vi "Auton Builder.vi"() -> ()   [LabVIEW 2017]
uses:
  Typedef/Field Settings.ctl
  Typedef/Robot Settings.ctl
  Typedef/Single Sequence.ctl
  Typedef/Sequence Command.ctl
  Typedef/Plate Arrangement.ctl
  Typedef/String Commands.ctl
  <vilib>/Utility/miscctls.llb/LVRowAndColumnTypeDef.ctl
  <vilib>/Analysis/coordinate.llb/2D Cartesian Coordinate Rotation (Array).vi
  <vilib>/Analysis/coordinate.llb/2D Cartesian Coordinate Shift (Array).vi
  <vilib>/Rock Robotics/Network Tables/NT Write Variant.vi
  <vilib>/Analysis/NI_AALPro.lvlib
panel:
  in  "Stop?":bool
  in  "Tab Control":enum32{"Builder", "Raw Sequence", "Settings"}(tab)
  in  "Index?":i32
  out "Issue:":string
  in  "Drive Time":bool
  in  "Other Commands":T1
  out "Current Command":string
  in  "Open":bool
  in  "Save":bool
  in  "Reset":bool
  out "Sequence Ok?":bool
  in  "Send to Robot":bool
  in  "Simulate":bool
  in  "Drive Path":bool
  in  "Turn Degrees":bool
  in  "Sequence Number":u32
  in  "Name":string
  in  "Plate Arrangement":T2={"LR*"=TRUE, "LL*"=TRUE, "RL*"=TRUE, "RR*"=TRUE}
  in  "Add":bool
  in  "Sequence":i32(listbox)
  in  "Right":bool
  in  "Mid":bool
  in  "Left":bool
  out "Field Half":cluster{dbl[], dbl[]}[](graph)
  in  "Cancel":bool
  in  "Auton Sequence":T3[](array[typedef])
  in  "Path Folder":path
  in  "Robot IP":string="roboRIO-3005-FRC.local"
  out "Connected?":bool
  in  "Field Settings":T5={"Exchange Left"=102.0, "Exchange Right"=150.0, "Power Cube Zone Left"=139.5, "Power Cube Zone Right"=139.5, "Switch Left"=85.25, "Switch Right"=85.25, "Switch Front"=140.0, "Switch Back"=196.0, "Platform Left"=95.25, "Platform Right"=95.25, "Platform Front"=261.47, "Slalom Depth"=235.235}
  in  "Robot Settings":T6={"Width"=34.0, "Length"=39.0} caption="Robot Settings w/ Bumpers"
  # "LEFT"
  # "FAR"
  # "NEAR"
  # "RIGHT"
  # "Commands"
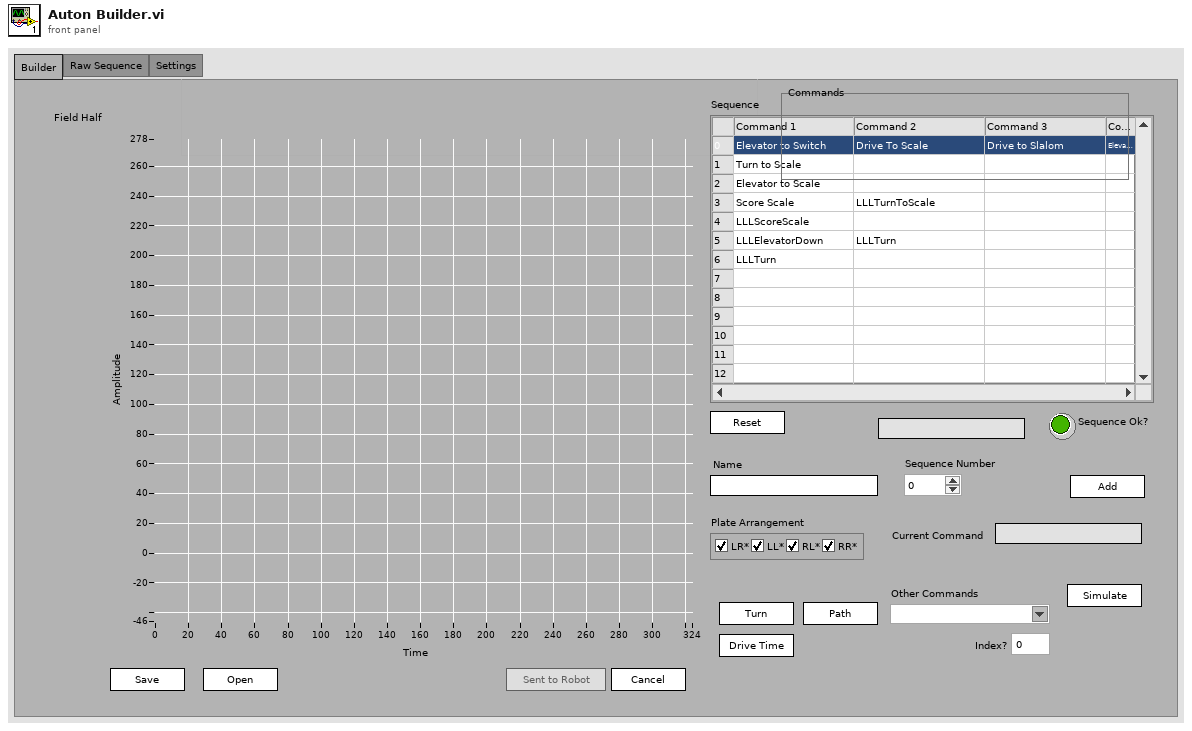
[diagram p1: front panel]
types:
  T1 = typedef "String Commands.ctl" = string
  T2 = typedef "Plate Arrangement.ctl" = cluster{"LR*":bool, "LL*":bool, "RL*":bool, "RR*":bool}
  T3 = typedef "Single Sequence.ctl" = cluster{"Sequence Array":T4[]}
  T4 = typedef "Sequence Command.ctl" = cluster{"Sequence Name":string, "Plate Arrangement":T2, "Command Name":string, "Data":variant, "Sequence Number":u32}
  T5 = typedef "Field Settings.ctl" = cluster{"Exchange Left":dbl, "Exchange Right":dbl, "Power Cube Zone Left":dbl, "Power Cube Zone Right":dbl, "Switch Left":dbl, "Switch Right":dbl, "Switch Front":dbl, "Switch Back":dbl, "Platform Left":dbl, "Platform Right":dbl, "Platform Front":dbl, "Slalom Depth":dbl}
  T6 = typedef "Robot Settings.ctl" = cluster{"Width":dbl, "Length":dbl}
  T7 = typedef "LVRowAndColumnTypeDef.ctl" = cluster{"Row":i32, "Column":i32}
  T8 = cluster{"Auton Sequence":T3[], "Field Half":cluster{dbl[], dbl[]}[], "Current Command":T4, "Robot Position":cluster{"x":dbl, "y":dbl}, "Theta":dbl, "y position":dbl, "Active Cell":T7, "Robot Index":i32, "Sequence OK?":bool, "Start Position":cluster{"x":dbl, "y":dbl}, "Field Selection":string, "Simulation Index":i32, "Sim Robot Index":i32, "Active Path":path, "Load Index":i32, "Graph Index":i32}
  T9 = typedef "LVPoint32TypeDef.ctl" = cluster{"Horizontal":i32, "Vertical":i32}
  T10 = cluster{"Shift":bool, "Ctrl":bool, "Alt":bool, "Cmd":bool, "Opt":bool}
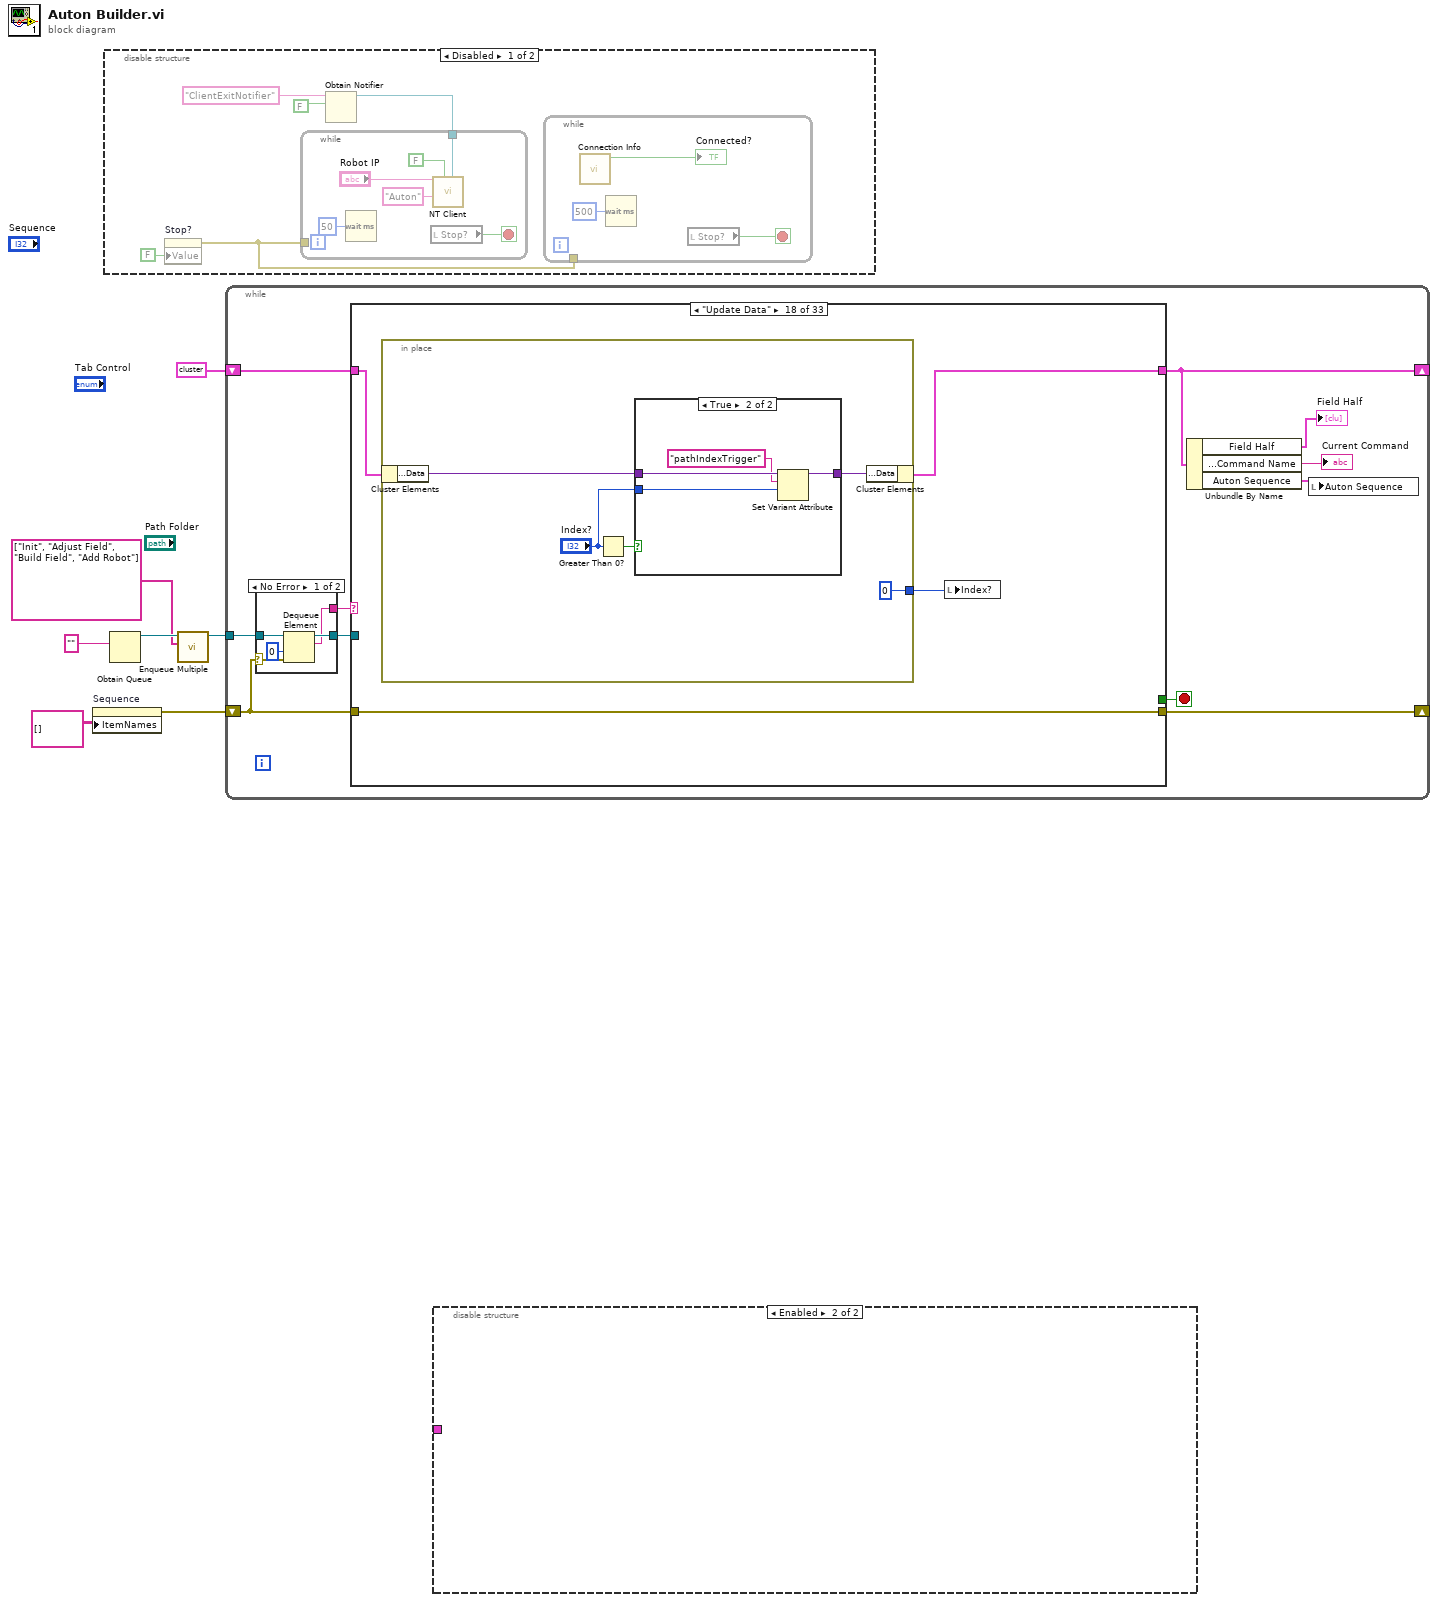
[diagram p0: block diagram]
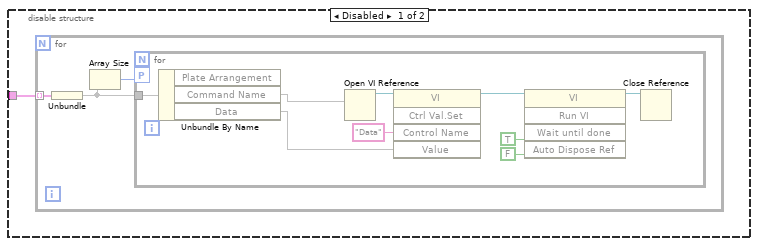
[diagram p3: hidden frame]
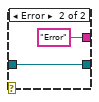
[diagram p4: hidden frame]
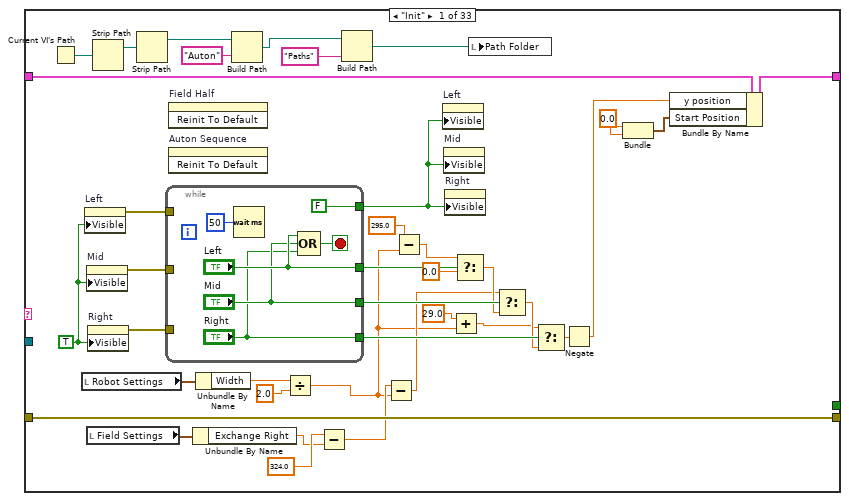
[diagram p5: hidden frame]
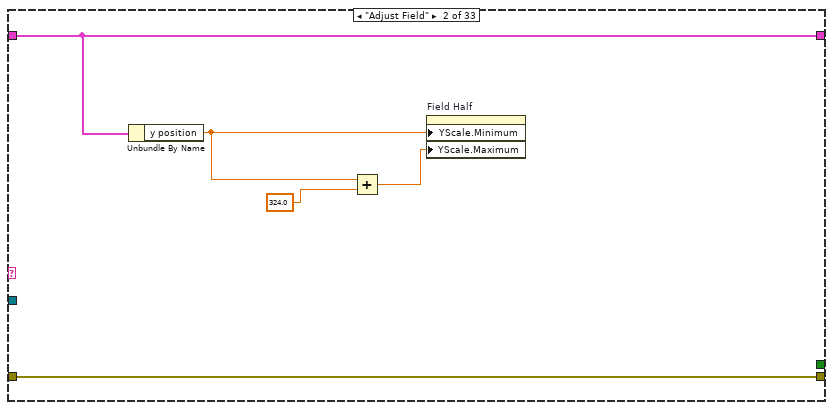
[diagram p6: hidden frame]
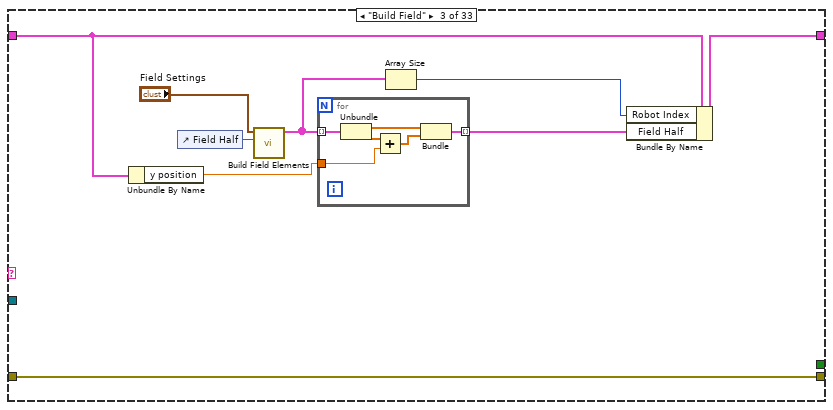
[diagram p7: hidden frame]
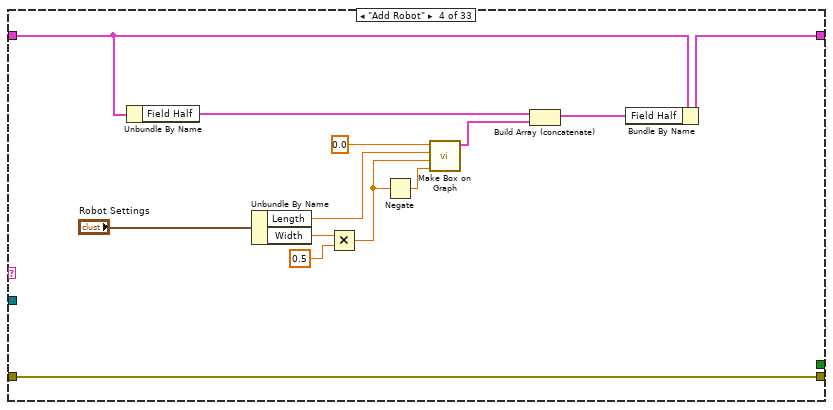
[diagram p8: hidden frame]
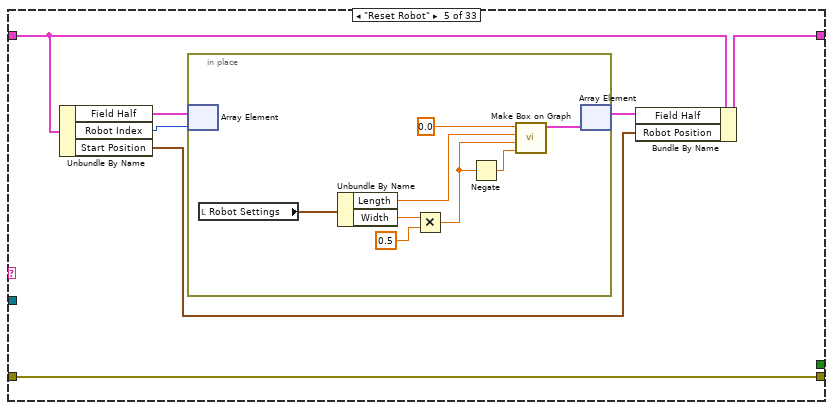
[diagram p9: hidden frame]
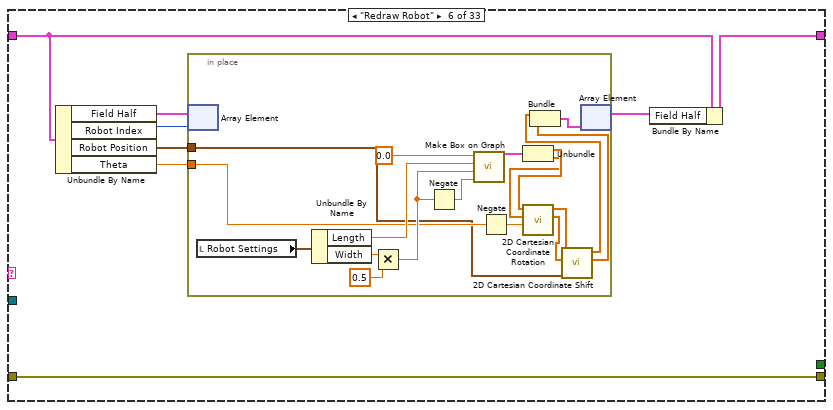
[diagram p10: hidden frame]
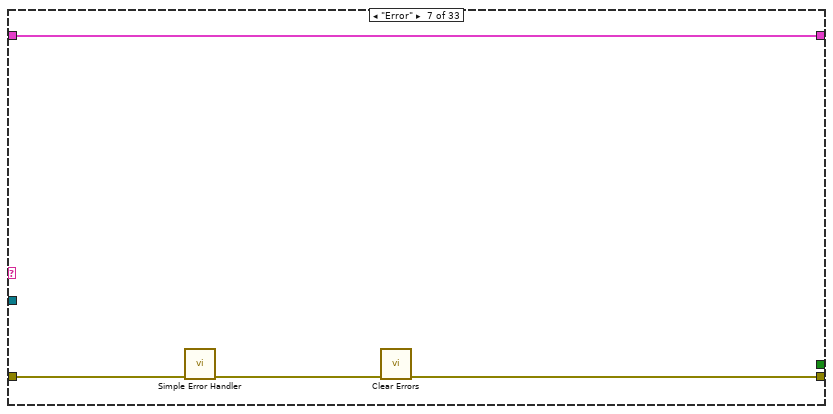
[diagram p11: hidden frame]
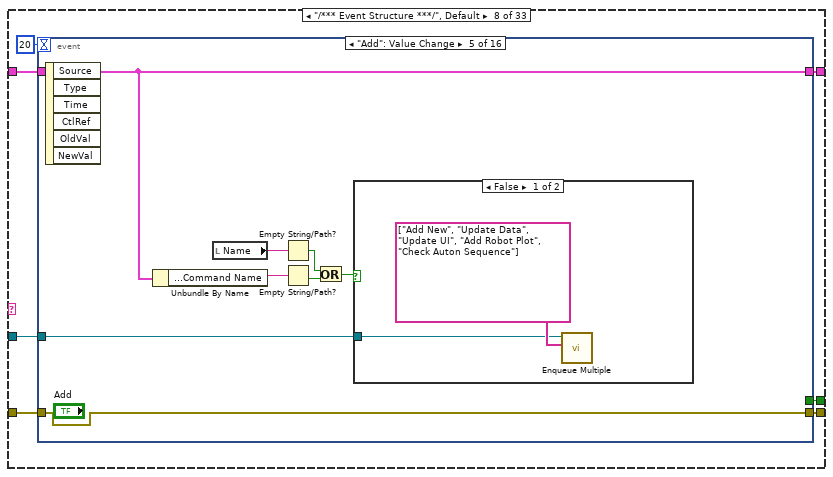
[diagram p12: hidden frame]
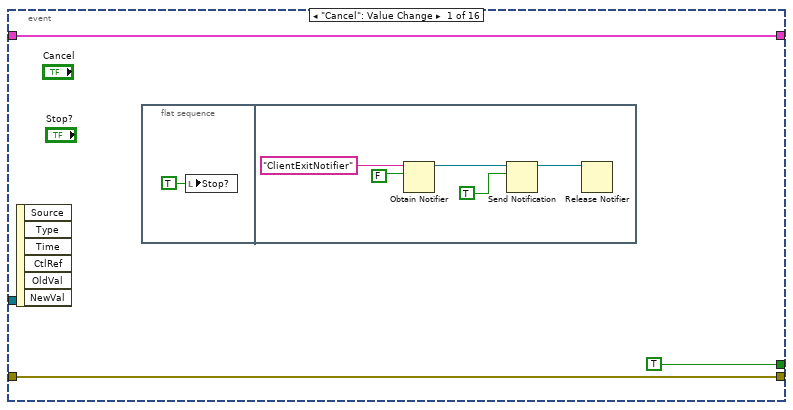
[diagram p13: hidden frame]
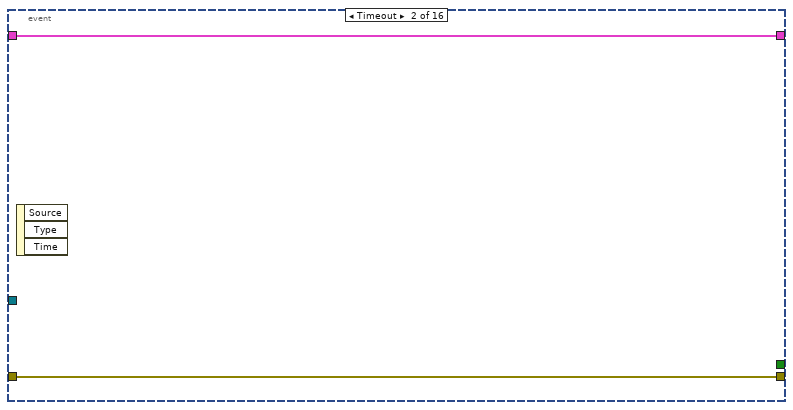
[diagram p14: hidden frame]
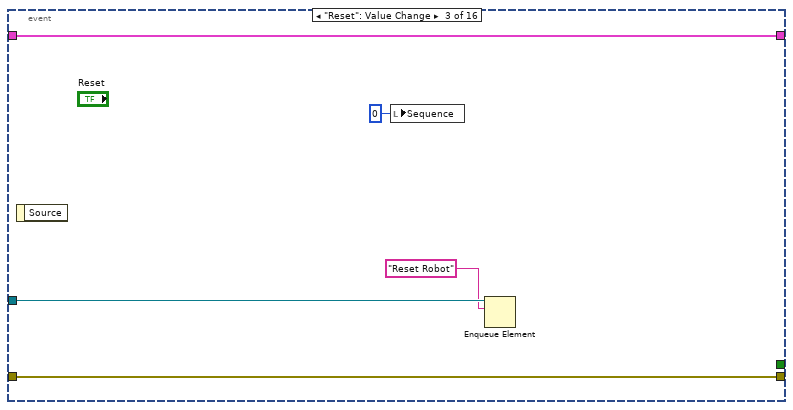
[diagram p15: hidden frame]
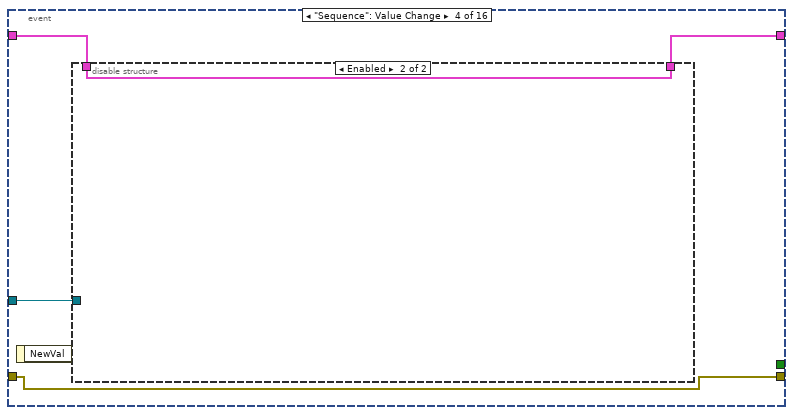
[diagram p16: hidden frame]
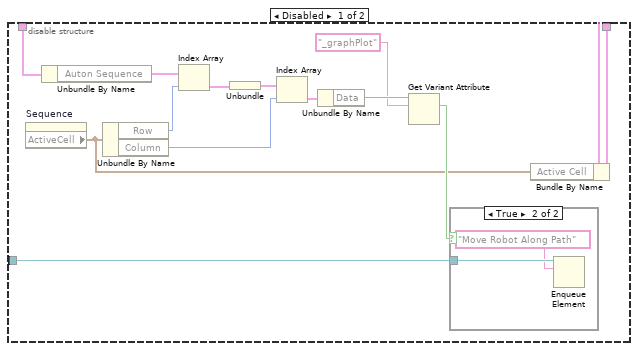
[diagram p17: hidden frame]
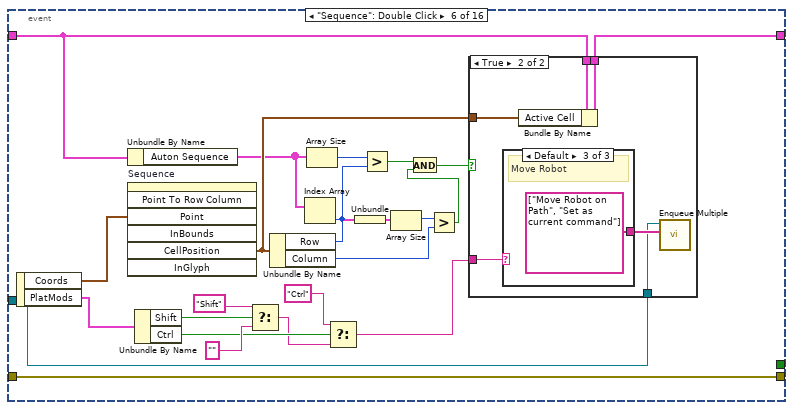
[diagram p20: hidden frame]
diagram:
  n1 = property on="Sequence" class="MCListbox (strict)"("ItemNames"=string[][] [] ("Item Names")) -> (error out=w7:errorcluster)  [unwired: 2 in, 1 out]
  n2 = disable-structure shown="Disabled" {
    frame Disabled {
      n3 = property on="Stop?" class="Bool (strict)"("Value"=FALSE ("Stop?")) -> (error out=w12:errorcluster)  [unwired: 2 in, 1 out]
      n4 = Obtain Notifier(name (unnamed)="ClientExitNotifier", notification data type=FALSE ("Automatic restart")) -> (notifier out=w9:refnum<notifier>)  [unwired: 2 in, 2 out]
      n5 = while {
        tunnel: w9 -> [w20]
        tunnel: w12 -> [_]
        stop <- w17 stop-if-true
        n6 = Wait (ms)(milliseconds to wait=u32 50) -> ()  [unwired: 1 out]
        n7 = local read "Stop?"() -> (w17:bool)
        n8 = call <vilib>:"NT Client.vi"("Cancel Ref"=w20, "Automatic restart"=FALSE, "Client Name"="Auton", "Server IP Address"="Robot IP") -> ()  [unwired: 8 in]
      }
      n9 = while {
        tunnel: w12 -> [_]
        stop <- w13 stop-if-true
        n10 = call <vilib>:"Connection Info.vi"() -> ("Connected"=→"Connected?":bool)  [unwired: 10 in, 1 out]
        n11 = Wait (ms)(milliseconds to wait=u32 500) -> ()  [unwired: 1 out]
        n12 = local read "Stop?"() -> (w13:bool)
      }
    }
    frame Enabled {
    }
  }
  n13 = Obtain Queue(element data type="") -> (queue out=w4:refnum<queue>)  [unwired: 4 in, 2 out]
  n14 = call "Enqueue Multiple.vi"("Array"=string[] ["Init", "Adjust Field", "Build Field", "Add Robot"], "Queue in"=w4) -> ("Queue out"=w3:refnum<queue>)  [unwired: 8 in, 1 out]
  n15 = while {
    shift-right: [w26] -> _
    shift-left: T8 {"Auton Sequence"=[], "Field Half"=[], "Current Command"={"Sequence Name"="", "Plate Arrangement"={"LR*"=FALSE, "LL*"=FALSE, "RL*"=FALSE, "RR*"=FALSE}, "Command Name"="", "Data"=variant, "Sequence Number"=0}, "Robot Position"={"x"=0.0, "y"=0.0}, "Theta"=0.0, "y position"=0.0, "Active Cell"={"Row"=0, "Column"=0}, "Robot Index"=0, "Sequence OK?"=FALSE, "Start Position"={"x"=0.0, "y"=0.0}, "Field Selection"="", "Simulation Index"=0, "Sim Robot Index"=0, "Active Path"=path "", "Load Index"=0, "Graph Index"=0} ("output cluster") -> [w32]
    shift-right: [w28] -> _
    shift-left: w7 -> [w27]
    tunnel: w3 -> [w31]
    stop <- w24 stop-if-true
    n16 = case shown="No Error" w27 {
      selector: w27 -> [w35 _]
      tunnel: w31 -> [w37 w39]
      tunnel: [w36 w39] -> w30
      tunnel: [w34 "Error"] -> w29
      frame No Error {
        n17 = Dequeue Element(queue=w37, timeout in ms (-1)=0, error in (no error)=w35) -> (queue out=w36:refnum<queue>, element=w34:string)  [unwired: 2 out]
      }
      frame Error {
      }
    }
    n18 = case shown="\"Update Data\"" w29 {
      tunnel: [_ _ _ _ _ _ _ w168 _ _ _ _ _ _ _ _ _ _ _ _ _ _ _ _ _ _ _ _ _ _ _ _ _] -> w24
      tunnel: w32 -> [w65 w87 w96 w106 w122 w138 w161 w167 w384 w402 w438 w456 w470 w483 w496 w513 w522 w541 w560 w575 w590 w632 w639 w646 w653 w655 w725 w739 w746 w758 w777 w791 w822]
      tunnel: [w64 w87 w94 w108 w123 w139 w161 w166 w382 w392 w428 w457 w471 w484 w497 w506 w519 w540 w554 w571 w589 w631 w639 w642 w651 w654 w720 w736 w746 w758 w773 w788 w822] -> w26
      tunnel: w30 -> [_ _ _ _ _ _ _ w165 _ w387 _ _ _ _ _ _ _ _ _ _ w582 _ _ w644 _ w658 w707 w732 _ _ w759 _ _]
      tunnel: [w63 w88 w92 w104 w121 w137 w160 w162 w385 w403 w439 w453 w468 w482 w494 w504 w523 w542 w556 w569 w594 w633 w638 w645 w652 w664 w726 w740 w745 w757 w760 w792 w824] -> w28
      tunnel: w27 -> [w63 w88 w92 w104 w121 w137 w159 w163 w385 w403 w439 w453 w468 w482 w494 w504 w523 w542 w556 w569 w594 w633 w638 w645 w652 w664 w726 w740 w745 w756 w772 w792 w824]
      frame "Init" {
        w52 = 0.0 ("f")
        w70 = TRUE ("Visible")
        n19 = Current VI's Path() -> (path=w46:path)
        n20 = local read "Robot Settings"() -> (w62:T6)
        n21 = property on="Left" class="Bool"("Visible"=w70) -> (error out=w72:errorcluster)  [unwired: 2 in, 1 out]
        n22 = property on="Mid" class="Bool"("Visible"=w70) -> (error out=w73:errorcluster)  [unwired: 2 in, 1 out]
        n23 = local read "Field Settings"() -> (w59:T5)
        n24 = property on="Right" class="Bool"("Visible"=w70) -> (error out=w71:errorcluster)  [unwired: 2 in, 1 out]
        n25 = Strip Path(path=w46) -> (stripped path=w45:path)  [unwired: 1 out]
        n26 = Strip Path(path=w45) -> (stripped path=w44:path)  [unwired: 1 out]
        n27 = while {
          tunnel: ["Left"] -> w75
          tunnel: ["Mid"] -> w76
          tunnel: ["Right"] -> w77
          tunnel: w73 -> [_]
          tunnel: w72 -> [_]
          tunnel: w71 -> [_]
          tunnel: [FALSE ("Visible")] -> w66
          stop <- w83 stop-if-true
          n28 = Wait (ms)(milliseconds to wait=u32 50) -> ()  [unwired: 1 out]
          n29 = Compound Arithmetic op=OR("Left", "Mid", "Right") -> (w83:bool)
        }
        n30 = invoke on="Field Half" class="XYGraph (strict)" method="Reinit To Default"() -> ()  [unwired: 3 in, 3 out]
        n31 = invoke on="Auton Sequence" class="Arr (strict)" method="Reinit To Default"() -> ()  [unwired: 3 in, 3 out]
        n32 = Unbundle By Name(w59) -> ("Exchange Right"=w56:dbl)
        n33 = Unbundle By Name(w62) -> ("Width"=w61:dbl)
        n34 = Build Path(base path=w44, name or relative path="Auton") -> (appended path=w42:path)
        n35 = Divide(x=w61, y=2.0) -> (x/y=w50:dbl)
        n36 = Subtract(x=324.0, y=w56) -> (x-y=w55:dbl)
        n37 = Build Path(base path=w42, name or relative path="Paths") -> (appended path=w40:path)
        n38 = Subtract(x=w55, y=w50) -> (x-y=w58:dbl)
        n39 = Subtract(x=295.0 ("y"), y=w50) -> (x-y=w51:dbl)
        n40 = property on="Left" class="Bool"("Visible"=w66) -> ()  [unwired: 2 in, 2 out]
        n41 = property on="Mid" class="Bool"("Visible"=w66) -> ()  [unwired: 2 in, 2 out]
        n42 = property on="Right" class="Bool"("Visible"=w66) -> ()  [unwired: 2 in, 2 out]
        n43 = Add(x=29.0 ("y"), y=w50) -> (x+y=w47:dbl)
        n44 = Select(t=w51, s=w75, f=0.0) -> (s? t:f=w69:dbl)
        n45 = local write "Path Folder"(w40) -> ()
        n46 = Select(t=w58, s=w76, f=w69) -> (s? t:f=w68:dbl)
        n47 = Select(t=w47, s=w77, f=w68) -> (s? t:f=w74:dbl)
        n48 = Negate(x=w74) -> (-x=w54:dbl)
        n49 = Bundle("f"=w52, "f"=w52) -> (w53:cluster{"f":dbl, "f":dbl})  [unwired: 1 in]
        n50 = Bundle By Name(cluster=w65, "y position"=w54, "Start Position"=w53) -> (w64:T8)
      }
      frame "Adjust Field" {
        n51 = Unbundle By Name(w87) -> ("y position"=w84:dbl)
        n52 = Add(x=w84, y=324.0 ("x")) -> (x+y=w86:dbl)
        n53 = property on="Field Half" class="XYGraph (strict)"("YScale.Minimum"=w84, "YScale.Maximum"=w86) -> ()  [unwired: 2 in, 2 out]
      }
      frame "Build Field" {
        n54 = Unbundle By Name(w96) -> ("y position"=w95:dbl)
        n55 = control-ref of="Field Half"() -> (w97:refnum<vi>)
        n56 = call "Build Field Elements.vi"("Field Half Graph"=w97, "Field Settings"="Field Settings") -> ("Field Half"=w91:cluster{dbl[], dbl[]}[])  [unwired: 9 in]
        n57 = for {
          tunnel: w91 -> [w103] mode=indexing
          tunnel: [w101] -> w93 mode=indexing
          tunnel: w95 -> [w98]
          n58 = Unbundle(w103) -> (w100:dbl[], w102:dbl[])
          n59 = Add(x=w102, y=w98) -> (x+y=w99:dbl[])
          n60 = Bundle(w100, w99) -> (w101:cluster{dbl[], dbl[]})  [unwired: 1 in]
        }
        n61 = Array Size(array=w91) -> (size(s)=w90:i32)
        n62 = Bundle By Name(cluster=w96, "Robot Index"=w90, "Field Half"=w93) -> (w94:T8)
      }
      frame "Add Robot" {
        n63 = Unbundle By Name(w106) -> ("Field Half"=w105:cluster{dbl[], dbl[]}[])
        n64 = Unbundle By Name("Robot Settings") -> ("Length"=w110:dbl, "Width"=w114:dbl)
        n65 = Multiply(x=w114, y=0.5 ("x")) -> (x*y=w112:dbl)
        n66 = Negate(x=w112) -> (-x=w111:dbl)
        n67 = call "Make Box on Graph.vi"("Y2"=w111, "Y1"=w112, "X2"=w110, "X1"=0.0) -> ("Output Graph"=w116:cluster{dbl[], dbl[]})  [unwired: 7 in]
        n68 = Build Array (concatenate)(w105, w116) -> (w107:cluster{dbl[], dbl[]}[])
        n69 = Bundle By Name(cluster=w106, "Field Half"=w107) -> (w108:T8)
      }
      frame "Reset Robot" {
        n70 = Unbundle By Name(w122) -> ("Field Half"=w120:cluster{dbl[], dbl[]}[], "Robot Index"=w119:i32, "Start Position"=w117:cluster{"x":dbl, "y":dbl})
        n71 = in-place {
          n72 = in-place-array #1(w120, w119) -> ()  [unwired: 1 out]
          n73 = local read "Robot Settings"() -> (w125:T6)
          n74 = Unbundle By Name(w125) -> ("Length"=w127:dbl, "Width"=w131:dbl)
          n75 = Multiply(x=w131, y=0.5 ("x")) -> (x*y=w129:dbl)
          n76 = Negate(x=w129) -> (-x=w128:dbl)
          n77 = call "Make Box on Graph.vi"("Y2"=w128, "Y1"=w129, "X2"=w127, "X1"=0.0) -> ("Output Graph"=w124:cluster{dbl[], dbl[]})  [unwired: 7 in]
          n78 = in-place-array #1(w124) -> (w118:cluster{dbl[], dbl[]}[])  [unwired: 1 out]
        }
        n79 = Bundle By Name(cluster=w122, "Field Half"=w118, "Robot Position"=w117) -> (w123:T8)
      }
      frame "Redraw Robot" {
        n80 = Unbundle By Name(w138) -> ("Field Half"=w136:cluster{dbl[], dbl[]}[], "Robot Index"=w135:i32, "Robot Position"=w133:cluster{"x":dbl, "y":dbl}, "Theta"=w132:dbl)
        n81 = in-place {
          in-place-border: w133 -> [w144]
          in-place-border: w132 -> [w147]
          n82 = in-place-array #2(w136, w135) -> ()  [unwired: 1 out]
          n83 = local read "Robot Settings"() -> (w151:T6)
          n84 = Unbundle By Name(w151) -> ("Length"=w153:dbl, "Width"=w157:dbl)
          n85 = Multiply(x=w157, y=0.5 ("x")) -> (x*y=w155:dbl)
          n86 = Negate(x=w155) -> (-x=w154:dbl)
          n87 = call "Make Box on Graph.vi"("Y2"=w154, "Y1"=w155, "X2"=w153, "X1"=0.0) -> ("Output Graph"=w150:cluster{dbl[], dbl[]})  [unwired: 7 in]
          n88 = Negate(x=w147) -> (-x=w140:dbl)
          n89 = Unbundle(w150) -> (w149:dbl[], w148:dbl[])
          n90 = call-poly <vilib>:"2D Cartesian Coordinate Rotation.vi"("theta"=w140, "Y"=w148, "X"=w149) -> ("Y Out"=w145:dbl[], "X Out"=w146:dbl[])  [unwired: 6 in, 1 out]
          n91 = call-poly <vilib>:"2D Cartesian Coordinate Shift.vi"("shift"=w144, "Y"=w145, "X"=w146) -> ("Y Out"=w142:dbl[], "X Out"=w143:dbl[])  [unwired: 6 in, 1 out]
          n92 = Bundle("X Out"=w143, "Y Out"=w142) -> (w141:cluster{"X Out":dbl[], "Y Out":dbl[]})  [unwired: 1 in]
          n93 = in-place-array #2(w141) -> (w134:cluster{dbl[], dbl[]}[])  [unwired: 1 out]
        }
        n94 = Bundle By Name(cluster=w138, "Field Half"=w134) -> (w139:T8)
      }
      frame "Error" {
        n95 = call <vilib>:"Simple Error Handler.vi"("error in (no error)"=w159) -> ("error out"=w158:errorcluster)  [unwired: 4 in, 4 out]
        n96 = call <vilib>:"Clear Errors.vi"("error in (no error)"=w158) -> ("error out"=w160:errorcluster)  [unwired: 5 in, 1 out]
      }
      frame "/*** Event Structure ***/", Default {
        n97 = event shown="[4] \"Add\": Value Change" {
          selector: _ -> [_ _ _ _ _ _ _ _ _ _ _ _ _ _ _ _]
          dyn-events: _ -> [_ _ _ _ _ _ _ _ _ _ _ _ _ _ _ _]
          timeout: 20 -> [_ _ _ _ _ _ _ _ _ _ _ _ _ _ _ _]
          tunnel: [TRUE _ _ _ _ _ _ _ _ _ _ _ _ _ _ _] -> w168
          tunnel: w167 -> [w170 w179 w184 w188 w212 w226 w270 w291 w299 w313 w317 w321 w328 w337 w343 w366]
          tunnel: [w170 w179 w184 w186 w212 w237 w269 w290 w298 w312 w316 w321 w328 w337 w342 w365] -> w166
          tunnel: w165 -> [_ _ w183 w187 w206 w224 _ _ w295 _ _ _ _ w335 w345 w368]
          tunnel: w163 -> [w169 w178 w180 w185 w205 w223 w258 w292 w297 w314 w318 w319 w327 w334 w346 w369]
          tunnel: [w169 w178 w180 w185 w205 w223 w258 w292 w296 w314 w318 w319 w327 w334 w340 w363] -> w162
          event "Cancel": Value Change {
            n98 = event-data() -> ()  [unwired: 1 in, 6 out]
            n99 = flat-sequence {
              frame #0 {
                n100 = local write "Stop?"(TRUE ("Stop?")) -> ()
              }
              frame #1 {
                n101 = Obtain Notifier(name (unnamed)="ClientExitNotifier", notification data type=FALSE ("Automatic restart")) -> (notifier out=w175:refnum<notifier>)  [unwired: 2 in, 2 out]
                n102 = Send Notification(notification=TRUE, notifier=w175) -> (notifier out=w173:refnum<notifier>)  [unwired: 1 in, 1 out]
                n103 = Release Notifier(notifier=w173) -> ()  [unwired: 2 in, 3 out]
              }
            }
          }
          event Timeout {
            n104 = event-data() -> ()  [unwired: 1 in, 3 out]
          }
          event "Reset": Value Change {
            n105 = event-data() -> ()  [unwired: 1 in, 1 out]
            n106 = local write "Sequence"(0 ("Sequence")) -> ()
            n107 = Enqueue Element(queue=w183, element="Reset Robot") -> ()  [unwired: 2 in, 3 out]
          }
          event "Sequence": Value Change {
            n108 = event-data() -> ()  [unwired: 1 in, 1 out]
            n109 = disable-structure shown="Enabled" {
              disable-tunnel: w188 -> [w201 w204]
              disable-tunnel: w187 -> [w192 _]
              disable-tunnel: [w190 w204] -> w186
              frame Disabled {
                n110 = property on="Sequence" class="MCListbox (strict)"() -> ("ActiveCell"=w189:T7)  [unwired: 2 in, 2 out]
                n111 = Unbundle By Name(w201) -> ("Auton Sequence"=w199:T3[])
                n112 = Unbundle By Name(w189) -> ("Row"=w200:i32, "Column"=w196:i32)
                n113 = Index Array(array=w199, index=w200) -> (element=w198:T3)
                n114 = Unbundle(w198) -> ("Sequence Array"=w197:T4[])
                n115 = Index Array(array=w197, index=w196) -> (element=w195:T4)
                n116 = Unbundle By Name(w195) -> ("Data"=w194:variant)
                n117 = Get Variant Attribute(Variant=w194, name="_graphPlot") -> (found=w191:bool)  [unwired: 2 in, 3 out]
                n118 = case shown="True" w191 {
                  tunnel: w192 -> [_ w203]
                  frame False {
                  }
                  frame True {
                    n119 = Enqueue Element(queue=w203, element="Move Robot Along Path") -> ()  [unwired: 2 in, 3 out]
                  }
                }
                n120 = Bundle By Name(cluster=w201, "Active Cell"=w189) -> (w190:T8)
              }
              frame Enabled {
              }
            }
          }
          event "Add": Value Change {
            n121 = event-data() -> ()  [unwired: 1 in, 6 out]
            n122 = Unbundle By Name(w212) -> ("Current Command.Command Name"=w211:string)
            n123 = local read "Name"() -> (w207:string)
            n124 = Empty String/Path?(string/path=w207) -> (empty?=w209:bool)
            n125 = Empty String/Path?(string/path=w211) -> (empty?=w210:bool)
            n126 = Or(x=w209, y=w210) -> (x .or. y?=w208:bool)
            n127 = case shown="False" w208 {
              tunnel: w206 -> [w213 _]
              frame False {
                n128 = call "Enqueue Multiple.vi"("Array"=string[] ["Add New", "Update Data", "Update UI", "Add Robot Plot", "Check Auton Sequence"], "Queue in"=w213) -> ()  [unwired: 8 in, 2 out]
              }
              frame True {
              }
            }
          }
          event "Sequence": Double Click {
            n129 = event-data() -> ("Coords"=w238:T9, "PlatMods"=w222:T10)  [unwired: 1 in]
            n130 = Unbundle By Name(w226) -> ("Auton Sequence"=w225:T3[])
            n131 = invoke on="Sequence" class="MCListbox (strict)" method="Point To Row Column"("Point"=w238) -> ("CellPosition"=w236:T7)  [unwired: 6 in, 6 out]
            n132 = Unbundle By Name(w222) -> ("Shift"=w221:bool, "Ctrl"=w218:bool)
            n133 = Select(t="Shift", s=w221, f="") -> (s? t:f=w216:string)
            n134 = Unbundle By Name(w236) -> ("Row"=w232:i32, "Column"=w228:i32)
            n135 = Index Array(array=w225, index=w232) -> (element=w231:T3)
            n136 = Array Size(array=w225) -> (size(s)=w235:i32)
            n137 = Select(t="Ctrl", s=w218, f=w216) -> (s? t:f=w217:string)
            n138 = Unbundle(w231) -> ("Sequence Array"=w230:T4[])
            n139 = Greater?(x=w235, y=w232) -> (0:w234:bool)
            n140 = Array Size(array=w230) -> (size(s)=w229:i32)
            n141 = Greater?(x=w229, y=w228) -> (0:w227:bool)
            n142 = And(x=w234, y=w227) -> (x .and. y?=w233:bool)
            n143 = case shown="True" w233 {
              tunnel: w226 -> [w239 w245]
              tunnel: [w239 w244] -> w237
              tunnel: w236 -> [_ w243]
              tunnel: w224 -> [_ w241]
              tunnel: w217 -> [_ w240]
              frame False {
              }
              frame True {
                n144 = case shown="Default" w240 {
                  tunnel: [string[] ["Prepare Delete", "Handle Graph Delete", "Check Auton Sequence"] ("Array") string[] ["Prepare Edit", "Edit Path"] ("Array") string[] ["Move Robot on Path", "Set as current command"] ("Array")] -> w242
                  frame "Shift" {
                    # "Delete Element"
                  }
                  frame "Ctrl" {
                    # "Delete Element"
                  }
                  frame Default {
                    # "Move Robot"
                  }
                }
                n145 = Bundle By Name(cluster=w245, "Active Cell"=w243) -> (w244:T8)
                n146 = call "Enqueue Multiple.vi"("Array"=w242, "Queue in"=w241) -> ()  [unwired: 8 in, 2 out]
              }
            }
          }
          event "Drive Path": Value Change {
            w249 = FALSE
            w256 = "Waypoints" ("name")
            n147 = event-data() -> ()  [unwired: 1 in, 1 out]
            n148 = local read "Robot Settings"() -> (w261:T6)
            n149 = Unbundle By Name(w270) -> ("Robot Position"=w275:cluster{"x":dbl, "y":dbl}, "y position"=w276:dbl, "Field Half"=w262:cluster{dbl[], dbl[]}[], "Current Command.Data"=w257:variant)
            n150 = local read "Field Settings"() -> (w259:T5)
            n151 = case shown="True" w249 {
              tunnel: w257 -> [_ w281]
              tunnel: cluster{dbl[], dbl[]} {[], []} ("value") -> [w277 w280]
              tunnel: w256 -> [_ w279]
              tunnel: [w277 w278] -> w255
              frame False {
              }
              frame True {
                n152 = Get Variant Attribute(Variant=w281, name=w279, default value (empty Variant)=w280) -> (value=w278:cluster{dbl[], dbl[]})  [unwired: 1 in, 3 out]
              }
            }
            n153 = Unbundle By Name(w261) -> ("Width"=w260:dbl)
            n154 = call "Path Builder.vi"("Edit? (F)"=w249, "Waypoints"=w255, "Field Settings"=w259, "Robot width (in)"=w260, "y start"=w276, "Start Point"=w275, "Field"=w262) -> ("Reverse Path?"=w252:bool, "Waypoints"=w263:cluster{dbl[], dbl[]}, "Graph Path"=w264:cluster{dbl[], dbl[]}, "Path"=w274:cluster{"x":dbl, "y":dbl}[])  [unwired: 1 in]
            n155 = Array Size(array=w262) -> (size(s)=w272:i32)
            n156 = To Variant(anything=w274) -> (Variant=w266:variant)
            n157 = Set Variant Attribute(Variant=w266, name="_graphPlot", value=w264) -> (Variant out=w267:variant)  [unwired: 1 in, 2 out]
            n158 = Set Variant Attribute(Variant=w267, name="_graphIndex", value=w272) -> (Variant out=w271:variant)  [unwired: 1 in, 2 out]
            n159 = Set Variant Attribute(Variant=w271, name=w256, value=w263) -> (Variant out=w253:variant)  [unwired: 1 in, 2 out]
            n160 = Set Variant Attribute(Variant=w253, name="reverse" ("Current Command.Command Name"), value=w252) -> (Variant out=w250:variant)  [unwired: 1 in, 2 out]
            n161 = Bundle By Name(cluster=w270, "Current Command.Data"=w250, "Current Command.Command Name"="Drive Path") -> (w269:T8)
          }
          event "Drive Time": Value Change {
            n162 = event-data() -> ()  [unwired: 1 in, 6 out]
            n163 = call "Drive for time"() -> ("Time (ms)"=w282:dbl, "Magnitude [1,-1]"=w283:dbl)  [unwired: 16 in, 2 out]
            n164 = Set Variant Attribute(Variant=variant, name="magnitude", value=w283) -> (Variant out=w288:variant)  [unwired: 1 in, 2 out]
            n165 = Set Variant Attribute(Variant=w288, name="time", value=w282) -> (Variant out=w285:variant)  [unwired: 1 in, 2 out]
            n166 = Bundle By Name(cluster=w291, "Current Command.Command Name"="Drive for Time" ("name"), "Current Command.Data"=w285) -> (w290:T8)
          }
          event "Auton Sequence": Value Change {
            n167 = event-data() -> ("NewVal"=w294:T3[])  [unwired: 1 in]
            n168 = Bundle By Name(cluster=w299, "Auton Sequence"=w294) -> (w298:T8)
            n169 = call "Enqueue Multiple.vi"("error in (no error)"=w297, "Array"=string[] ["Build Field", "Add Robot", "Reload Listbox", "Reload Graphs", "Check Auton Sequence"], "Queue in"=w295) -> ("error out"=w296:errorcluster)  [unwired: 7 in, 1 out]
          }
          event "Turn Degrees": Value Change {
            # "Default timeout = 3 seconds"
            n170 = event-data() -> ()  [unwired: 1 in, 1 out]
            n171 = call "Turn Angle Prompt"() -> ("Timeout (ms) 3000 = default"=w303:dbl, "Turn angle (degrees)"=w310:dbl)  [unwired: 16 in, 2 out]
            n172 = Equal To 0?(x=w303) -> (x = 0?=w304:bool)
            n173 = Select(t=3000.0, s=w304, f=w303) -> (s? t:f=w301:dbl)
            n174 = Set Variant Attribute(Variant=variant, name="angle", value=w310) -> (Variant out=w308:variant, error out=w309:errorcluster)  [unwired: 1 in, 1 out]
            n175 = Set Variant Attribute(Variant=w308, name="timeout", value=w301, error in=w309) -> (Variant out=w307:variant)  [unwired: 2 out]
            n176 = Bundle By Name(cluster=w313, "Current Command.Data"=w307, "Current Command.Command Name"="Turn Degrees" ("name")) -> (w312:T8)
          }
          event Value Change {
            n177 = event-data() -> ("NewVal"=w315:T1)  [unwired: 1 in]
            n178 = Bundle By Name(cluster=w317, "Current Command.Command Name"=w315) -> (w316:T8)
          }
          event "Send to Robot": Value Change {
            n179 = event-data() -> ()  [unwired: 1 in, 6 out]
            n180 = local read "Connected?"() -> (w320:bool)
            n181 = case shown="True" w320 {
              tunnel: w321 -> [_ w326]
              frame False {
                n182 = One Button Dialog(message="Must be connected to the robot to send to the robot!") -> ()  [unwired: 1 in, 1 out]
              }
              frame True {
                n183 = Unbundle By Name(w326) -> ("Auton Sequence"=w325:T3[])
                n184 = To Variant(anything=w325) -> (Variant=w324:variant)
                n185 = call-poly <vilib>:"NT Write Value.vi"("Variant"=w324, "Name"="AutonSequence_NT") -> ()  [unwired: 9 in, 1 out]
              }
            }
          }
          event "Robot IP": Value Change {
            n186 = event-data() -> ()  [unwired: 1 in, 6 out]
            n187 = Obtain Notifier(name (unnamed)="ClientExitNotifier", notification data type=FALSE ("Automatic restart")) -> (notifier out=w331:refnum<notifier>)  [unwired: 2 in, 2 out]
            n188 = Send Notification(notification=TRUE, notifier=w331) -> (notifier out=w329:refnum<notifier>)  [unwired: 1 in, 1 out]
            n189 = Release Notifier(notifier=w329) -> ()  [unwired: 2 in, 3 out]
          }
          event "Simulate": Value Change {
            n190 = event-data() -> ()  [unwired: 1 in, 1 out]
            n191 = call "Enqueue Multiple.vi"("Array"=string[] ["Check Auton Sequence", "Reset Robot", "Simulation Init"], "Queue in"=w335) -> ()  [unwired: 8 in, 2 out]
          }
          event "Save": Value Change {
            n192 = event-data() -> ()  [unwired: 1 in, 1 out]
            n193 = local read "Path Folder"() -> (w349:path)
            n194 = call "File Dialog"("start path"=w349, "error in"=w346, "pattern (all files)"="*.AUTONPATH", "pattern label"="FRC Auton Path") -> ("selected path"=w344:path, "exists"=w338:bool, "cancelled"=w341:bool, "error out"=w340:errorcluster)  [unwired: 8 in]
            n195 = Or(x=w341, y=w340) -> (x .or. y?=w339:bool)
            n196 = case shown="False" w339 {
              tunnel: w345 -> [w355 _]
              tunnel: w344 -> [w352 _]
              tunnel: w343 -> [w354 w361]
              tunnel: [w353 w361] -> w342
              tunnel: w338 -> [w350 _]
              frame False {
                n197 = case shown="False" w350 {
                  tunnel: [TRUE ("T button?") w358] -> w351
                  frame False {
                  }
                  frame True {
                    n198 = Two Button Dialog(message="Overwrite File?") -> (T button?=w358:bool)  [unwired: 2 in]
                  }
                }
                n199 = case shown="True" w351 {
                  tunnel: w355 -> [_ w360]
                  frame False {
                  }
                  frame True {
                    n200 = Enqueue Element(queue=w360, element="Save File") -> ()  [unwired: 2 in, 3 out]
                  }
                }
                n201 = Bundle By Name(cluster=w354, "Active Path"=w352) -> (w353:T8)
              }
              frame True {
              }
            }
          }
          event "Open": Value Change {
            n202 = event-data() -> ()  [unwired: 1 in, 1 out]
            n203 = local read "Path Folder"() -> (w372:path)
            n204 = call "File Dialog2"("start path"=w372, "error in"=w369, "pattern (all files)"="*.AUTONPATH", "pattern label"="FRC Auton Path") -> ("selected path"=w367:path, "cancelled"=w364:bool, "error out"=w363:errorcluster)  [unwired: 8 in, 1 out]
            n205 = Or(x=w364, y=w363) -> (x .or. y?=w362:bool)
            n206 = case shown="False" w362 {
              tunnel: w368 -> [w377 _]
              tunnel: w367 -> [w374 _]
              tunnel: w366 -> [w376 w378]
              tunnel: [w375 w378] -> w365
              frame False {
                n207 = Bundle By Name(cluster=w376, "Active Path"=w374) -> (w375:T8)
                n208 = Enqueue Element(queue=w377, element="Open File") -> ()  [unwired: 2 in, 3 out]
              }
              frame True {
              }
            }
          }
        }
      }
      frame "Check Auton Sequence" {
        # "#check robot position is contiguous as well"
        n209 = Unbundle By Name(w384) -> ("Auton Sequence"=w383:T3[])
        n210 = call "Validate Sequence.vi"("Auton Sequence"=w383) -> ("Command Name"=→"Issue:":string, "Sequence Ok?"=w380:bool)  [unwired: 9 in]
        "Sequence Ok?" <- w380
        n211 = Bundle By Name(cluster=w384, "Sequence OK?"=w380) -> (w382:T8)
        n212 = Not(x=w380) -> (.not. x?=w379:bool)
        n213 = property on="Issue:" class="Str"("Visible"=w379) -> ()  [unwired: 2 in, 2 out]
      }
      frame "Move Robot on Path" {
        n214 = Unbundle By Name(w402) -> ("Robot Index"=w390:i32, "Field Half"=w391:cluster{dbl[], dbl[]}[], "Auton Sequence"=w394:T3[], "Active Cell"=w393:T7)
        n215 = Unbundle By Name(w393) -> ("Row"=w401:i32, "Column"=w398:i32)
        n216 = Index Array(array=w391, index=w390) -> (element=w386:cluster{dbl[], dbl[]})
        n217 = Index Array(array=w394, index=w401) -> (element=w400:T3)
        n218 = Unbundle(w400) -> ("Sequence Array"=w399:T4[])
        n219 = Index Array(array=w399, index=w398) -> (element=w397:T4)
        n220 = Unbundle By Name(w397) -> ("Data"=w396:variant)
        n221 = Get Variant Attribute(Variant=w396, name="_graphPlot", default value (empty Variant)=w386) -> (found=w388:bool, value=w389:cluster{dbl[], dbl[]})  [unwired: 1 in, 2 out]
        n222 = case shown="True" w388 {
          tunnel: w402 -> [w404 w422]
          tunnel: [w404 w421] -> w392
          tunnel: w390 -> [_ _]
          tunnel: w389 -> [_ w408]
          tunnel: w387 -> [_ w410]
          frame False {
          }
          frame True {
            n223 = Unbundle(w408) -> (w414:dbl[], w415:dbl[])
            n224 = Array Size(array=w414) -> (size(s)=w413:i32)
            n225 = Decrement(x=w413) -> (x-1=w406:i32)
            n226 = Subtract(x=w406, y=5) -> (x-y=w405:i32)
            n227 = Array Subset(array=w414, index=w405) -> (w418:dbl[])  [unwired: 1 in]
            n228 = Array Subset(array=w415, index=w405) -> (w419:dbl[])  [unwired: 1 in]
            n229 = Index Array(array=w414, index=w406) -> (element=w417:dbl)
            n230 = Index Array(array=w415, index=w406) -> (element=w416:dbl)
            n231 = Bundle("x"=w417, "y"=w416) -> (w411:cluster{"x":dbl, "y":dbl})  [unwired: 1 in]
            n232 = call <vilib>:"Linear Fit.vi"("Y"=w419, "X"=w418) -> ("slope"=w420:dbl)  [unwired: 9 in, 4 out]
            n233 = Enqueue Element At Opposite End(queue=w410, element="Redraw Robot") -> ()  [unwired: 2 in, 3 out]
            n234 = Inverse Tangent(1:w420) -> (0:w412:dbl)
            n235 = Bundle By Name(cluster=w422, "Robot Position"=w411, "Theta"=w412) -> (w421:T8)
          }
        }
      }
      frame "Move Robot on Path Old" {
        n236 = Unbundle By Name(w438) -> ("Robot Index"=w426:i32, "Field Half"=w427:cluster{dbl[], dbl[]}[], "Auton Sequence"=w430:T3[], "Active Cell"=w429:T7)
        n237 = Unbundle By Name(w429) -> ("Row"=w437:i32, "Column"=w434:i32)
        n238 = Index Array(array=w427, index=w426) -> (element=w425:cluster{dbl[], dbl[]})
        n239 = Index Array(array=w430, index=w437) -> (element=w436:T3)
        n240 = Unbundle(w436) -> ("Sequence Array"=w435:T4[])
        n241 = Index Array(array=w435, index=w434) -> (element=w433:T4)
        n242 = Unbundle By Name(w433) -> ("Data"=w432:variant)
        n243 = Get Variant Attribute(Variant=w432, name="_graphPlot") -> (found=w423:bool, value=w424:variant)  [unwired: 2 in, 2 out]
        n244 = case shown="True" w423 {
          tunnel: w438 -> [w440 w450]
          tunnel: [w440 w449] -> w428
          tunnel: w427 -> [_ w448]
          tunnel: w426 -> [_ w445]
          tunnel: w425 -> [_ w444]
          tunnel: w424 -> [_ w442]
          frame False {
          }
          frame True {
            n245 = Variant To Data(type=w444, Variant=w442) -> (data=w446:cluster{dbl[], dbl[]})  [unwired: 1 in, 1 out]
            n246 = call "Move Robot to End of Path.vi"("Robot Path"=w446, "Robot Plot"=w444) -> ("Robot Position"=w441:cluster{"x":dbl, "y":dbl}, "Robot Plot Out"=w443:cluster{dbl[], dbl[]})  [unwired: 8 in]
            n247 = Replace Array Subset(array=w448, new element=w443, index=w445) -> (w447:cluster{dbl[], dbl[]}[])
            n248 = Bundle By Name(cluster=w450, "Field Half"=w447, "Robot Position"=w441) -> (w449:T8)
          }
        }
      }
      frame "Prepare Delete" {
        n249 = Unbundle By Name(w456) -> ("Auton Sequence"=w452:T3[], "Active Cell"=w455:T7)
        n250 = Unbundle By Name(w455) -> ("Row"=w460:i32, "Column"=w462:i32)
        n251 = Index Array(array=w452, index=w460) -> (element=w464:T3)
        n252 = Unbundle(w464) -> ("Sequence Array"=w463:T4[])
        n253 = Delete From Array(array=w463, length=1, index=w462) -> (array with subset deleted=w454:T4[])  [unwired: 1 out]
        n254 = Index Array(array=w463, index=w462) -> (element=w461:T4)
        n255 = Bundle("Sequence Array"=w454) -> (w459:cluster{"Sequence Array":T4[]})  [unwired: 1 in]
        n256 = flat-sequence {
          tunnel: w451 -> [w465]
          frame #0 {
            n257 = control-ref of="Sequence"() -> (w466:refnum<vi>)
            n258 = call "Update Table Display.vi"("Auton Sequence"=w465, "MulticolumnListbox in"=w466) -> ()  [unwired: 10 in]
          }
        }
        n259 = Replace Array Subset(array=w452, new element=w459, index=w460) -> (w451:T3[])
        n260 = Bundle By Name(cluster=w456, "Current Command"=w461, "Auton Sequence"=w451) -> (w457:T8)
      }
      frame "Prepare Edit" {
        n261 = Unbundle By Name(w470) -> ("Auton Sequence"=w467:T3[], "Active Cell"=w469:T7)
        n262 = Unbundle By Name(w469) -> ("Row"=w472:i32, "Column"=w474:i32)
        n263 = Index Array(array=w467, index=w472) -> (element=w476:T3)
        n264 = Unbundle(w476) -> ("Sequence Array"=w475:T4[])
        n265 = Index Array(array=w475, index=w474) -> (element=w473:T4)
        n266 = Bundle By Name(cluster=w470, "Current Command"=w473) -> (w471:T8)
      }
      frame "Update Edit Sequence" {
        n267 = Unbundle By Name(w483) -> ("Current Command"=w477:T4, "Auton Sequence"=w481:T3[], "Active Cell"=w479:T7)
        n268 = Unbundle By Name(w479) -> ("Row"=w478:i32)
        n269 = in-place {
          in-place-border: w479 -> [w491]
          in-place-border: w477 -> [w485]
          n270 = in-place-array #3(w481, w478) -> (w490:T3)
          n271 = Unbundle By Name(w491) -> ("Column"=w486:i32)
          n272 = Unbundle(w490) -> ("Sequence Array"=w489:T4[])
          n273 = in-place {
            in-place-border: w485 -> [w492]
            n274 = in-place-array #4(w489, w486) -> ()  [unwired: 1 out]
            n275 = in-place-array #4(w492) -> (w488:T4[])  [unwired: 1 out]
          }
          n276 = Bundle("Sequence Array"=w488) -> (w487:cluster{"Sequence Array":T4[]})  [unwired: 1 in]
          n277 = in-place-array #3(w487) -> (w480:T3[])  [unwired: 1 out]
        }
        n278 = Bundle By Name(cluster=w483, "Auton Sequence"=w480) -> (w484:T8)
      }
      frame "Set as current command" {
        n279 = Unbundle By Name(w496) -> ("Auton Sequence"=w493:T3[], "Active Cell"=w495:T7)
        n280 = Unbundle By Name(w495) -> ("Row"=w498:i32, "Column"=w500:i32)
        n281 = Index Array(array=w493, index=w498) -> (element=w502:T3)
        n282 = Unbundle(w502) -> ("Sequence Array"=w501:T4[])
        n283 = Index Array(array=w501, index=w500) -> (element=w499:T4)
        n284 = Bundle By Name(cluster=w496, "Current Command"=w499) -> (w497:T8)
      }
      frame "Handle Graph Delete" {
        n285 = Unbundle By Name(w513) -> ("Field Half"=w507:cluster{dbl[], dbl[]}[], "Current Command"=w512:T4)
        n286 = Unbundle By Name(w512) -> ("Data"=w511:variant)
        n287 = Get Variant Attribute(Variant=w511, name="_graphIndex", default value (empty Variant)=0) -> (found=w503:bool, value=w509:i32)  [unwired: 1 in, 2 out]
        n288 = case shown="True" w503 {
          tunnel: w509 -> [_ w517]
          tunnel: w507 -> [w514 w516]
          tunnel: [w514 w515] -> w505
          frame False {
          }
          frame True {
            n289 = in-place {
              n290 = in-place-array #5(w516, w517) -> ()  [unwired: 1 out]
              n291 = in-place-array #5(cluster{dbl[], dbl[]} {[], []} ("element")) -> (w515:cluster{dbl[], dbl[]}[])  [unwired: 1 out]
            }
          }
        }
        n292 = Bundle By Name(cluster=w513, "Field Half"=w505) -> (w506:T8)
      }
      frame "Add New" {
        w529 = T4 {"Sequence Name"="", "Plate Arrangement"={"LR*"=TRUE, "LL*"=TRUE, "RL*"=TRUE, "RR*"=TRUE}, "Command Name"="", "Data"=variant, "Sequence Number"=0}  # Current Command
        n293 = Unbundle By Name(w522) -> ("Auton Sequence"=w521:T3[])
        n294 = Initialize Array(w529) -> (w528:T4[])  [unwired: 1 in]
        n295 = Array Size(array=w521) -> (size(s)=w531:i32)
        n296 = Bundle(w528) -> (w527:cluster{T4[]})  [unwired: 1 in]
        n297 = Bundle By Name(cluster=w522, "Current Command.Sequence Number"="Sequence Number", "Current Command.Plate Arrangement"="Plate Arrangement", "Current Command.Sequence Name"="Name") -> (w520:T8)
        n298 = Greater Or Equal?(x="Sequence Number", y=w531) -> (x >= y?=w530:bool)
        n299 = case shown="True" w530 {
          tunnel: w521 -> [_ w538]
          tunnel: w527 -> [_ w537]
          tunnel: "Sequence Number" -> [_ w536]
          tunnel: w520 -> [w532 w535]
          tunnel: [w532 w533] -> w519
          frame False {
          }
          frame True {
            n300 = Insert Into Array(array=w538, index=w536, new element=w537) -> (w534:T3[])
            n301 = Bundle By Name(cluster=w535, "Auton Sequence"=w534) -> (w533:T8)
          }
        }
      }
      frame "Update Data" {
        n302 = in-place {
          in-place-border: [0] -> w539
          n303 = in-place-cluster #6(w541) -> ("Current Command.Data"=w547:variant)
          n304 = Greater Than 0?(x="Index?") -> (x > 0?=w545:bool)
          n305 = case shown="True" w545 {
            tunnel: w547 -> [w548 w552]
            tunnel: [w548 w551] -> w546
            tunnel: "Index?" -> [_ w549]
            frame False {
            }
            frame True {
              n306 = Set Variant Attribute(Variant=w552, name="pathIndexTrigger", value=w549) -> (Variant out=w551:variant)  [unwired: 1 in, 2 out]
            }
          }
          n307 = in-place-cluster #6("Current Command.Data"=w546) -> (w540:T8)
        }
        n308 = local write "Index?"(w539) -> ()
      }
      frame "Update UI" {
        n309 = Unbundle By Name(w560) -> ("Auton Sequence"=w555:T3[], "Current Command.Sequence Number"=w558:u32, "Current Command"=w559:T4)
        n310 = in-place {
          in-place-border: w559 -> [w565]
          n311 = in-place-array #7(w555, w558) -> (w563:T3)
          n312 = Unbundle(w563) -> ("Sequence Array"=w561:T4[])
          n313 = Build Array (concatenate)(w561, w565) -> (w564:T4[])
          n314 = Bundle(w564) -> (w562:cluster{T4[]})  [unwired: 1 in]
          n315 = in-place-array #7(w562) -> (w553:T3[])  [unwired: 1 out]
        }
        n316 = control-ref of="Sequence"() -> (w557:refnum<vi>)
        n317 = Bundle By Name(cluster=w560, "Auton Sequence"=w553) -> (w554:T8)
        n318 = call "Update Table Display.vi"("Auton Sequence"=w553, "MulticolumnListbox in"=w557) -> ()  [unwired: 10 in]
      }
      frame "Add Robot Plot" {
        n319 = Unbundle By Name(w575) -> ("Field Half"=w568:cluster{dbl[], dbl[]}[], "Current Command.Data"=w574:variant)
        n320 = Index Array(array=w568) -> (element=w566:cluster{dbl[], dbl[]})  [unwired: 1 in]
        n321 = Get Variant Attribute(Variant=w574, name="_graphPlot") -> (found=w572:bool, value=w567:variant)  [unwired: 2 in, 2 out]
        n322 = case shown="True" w572 {
          tunnel: [w576 w581] -> w570
          tunnel: w568 -> [w576 w580]
          tunnel: w567 -> [_ w579]
          tunnel: w566 -> [_ w578]
          frame False {
          }
          frame True {
            n323 = Variant To Data(type=w578, Variant=w579) -> (data=w577:cluster{dbl[], dbl[]})  [unwired: 1 in, 1 out]
            n324 = Build Array (concatenate)(w580, w577) -> (w581:cluster{dbl[], dbl[]}[])
          }
        }
        n325 = Bundle By Name(cluster=w575, "Field Half"=w570) -> (w571:T8)
      }
      frame "Edit Path" {
        n326 = Unbundle By Name(w590) -> ("Robot Position"=w592:cluster{"x":dbl, "y":dbl}, "y position"=w593:dbl, "Field Half"=w591:cluster{dbl[], dbl[]}[], "Current Command.Data"=w588:variant)
        n327 = Get Variant Attribute(Variant=w588, name="_graphIndex", default value (empty Variant)=0 ("size(s)")) -> (duplicate Variant=w587:variant, found=w584:bool, value=w583:i32)  [unwired: 1 in, 1 out]
        n328 = case shown="True" w584 {
          tunnel: w593 -> [_ w626]
          tunnel: w592 -> [_ w625]
          tunnel: w591 -> [_ w619]
          tunnel: w590 -> [w595 w607]
          tunnel: [w595 w606] -> w589
          tunnel: w587 -> [_ w600]
          tunnel: w583 -> [_ w598]
          tunnel: w582 -> [_ w597]
          frame False {
          }
          frame True {
            w609 = "Waypoints" ("name")
            n329 = local read "Robot Settings"() -> (w618:T6)
            n330 = local read "Field Settings"() -> (w616:T5)
            n331 = Unbundle By Name(w618) -> ("Width"=w617:dbl)
            n332 = Get Variant Attribute(Variant=w600, name="reverse" ("Current Command.Command Name"), default value (empty Variant)=FALSE) -> (duplicate Variant=w601:variant, value=w602:bool)  [unwired: 1 in, 2 out]
            n333 = Get Variant Attribute(Variant=w601, name=w609, default value (empty Variant)=cluster{dbl[], dbl[]} {[], []} ("value")) -> (value=w615:cluster{dbl[], dbl[]})  [unwired: 1 in, 3 out]
            n334 = call "Path Builder.vi"("Edit? (F)"=TRUE, "Reverse Path"=w602, "Waypoints"=w615, "Field Settings"=w616, "Robot width (in)"=w617, "y start"=w626, "Start Point"=w625, "Field"=w619) -> ("Reverse Path?"=w613:bool, "Waypoints"=w620:cluster{dbl[], dbl[]}, "Graph Path"=w621:cluster{dbl[], dbl[]}, "Path"=w624:cluster{"x":dbl, "y":dbl}[])
            n335 = To Variant(anything=w624) -> (Variant=w622:variant)
            n336 = Set Variant Attribute(Variant=w622, name="_graphPlot", value=w621) -> (Variant out=w623:variant)  [unwired: 1 in, 2 out]
            n337 = Set Variant Attribute(Variant=w623, name=w609, value=w620) -> (Variant out=w614:variant)  [unwired: 1 in, 2 out]
            n338 = Set Variant Attribute(Variant=w614, name="reverse" ("Current Command.Command Name"), value=w613) -> (Variant out=w612:variant)  [unwired: 1 in, 2 out]
            n339 = Bundle By Name(cluster=w607, "Current Command.Command Name"="Drive Path", "Current Command.Data"=w612, "Graph Index"=w598) -> (w606:T8)
            n340 = call "Enqueue Multiple.vi"("Array"=string[] ["Update Graph Index", "Update Edit Sequence"], "Queue in"=w597) -> ()  [unwired: 8 in, 2 out]
          }
        }
      }
      frame "Update Graph Index" {
        n341 = Unbundle By Name(w632) -> ("Field Half"=w630:cluster{dbl[], dbl[]}[], "Graph Index"=w629:i32, "Current Command.Data"=w628:variant)
        n342 = in-place {
          in-place-border: w628 -> [w636]
          n343 = in-place-array #8(w630, w629) -> ()  [unwired: 1 out]
          n344 = Get Variant Attribute(Variant=w636, name="_graphPlot", default value (empty Variant)=cluster{dbl[], dbl[]} {[], []} ("value")) -> (value=w634:cluster{dbl[], dbl[]})  [unwired: 1 in, 3 out]
          n345 = in-place-array #8(w634) -> (w627:cluster{dbl[], dbl[]}[])  [unwired: 1 out]
        }
        n346 = Bundle By Name(cluster=w632, "Field Half"=w627) -> (w631:T8)
      }
      frame "/**** Simulation Functions ****/" {
      }
      frame "Simulation Init" {
        n347 = local read "Sequence Ok?"() -> (w643:bool)
        n348 = case shown="True" w643 {
          tunnel: w644 -> [_ w648]
          frame False {
            n349 = One Button Dialog(message="Invalid Sequence, fix before running simulation") -> ()  [unwired: 1 in, 1 out]
          }
          frame True {
            n350 = call "Enqueue Multiple.vi"("Array"=string[] ["Select Field String", "Run Next Sequence", "Sequence Next"], "Queue in"=w648) -> ()  [unwired: 8 in, 2 out]
          }
        }
        n351 = Bundle By Name(cluster=w646, "Simulation Index"=0, "Sim Robot Index"=0) -> (w642:T8)
      }
      frame "Select Field String" {
        n352 = call "Prompt User for Input"() -> ("Field Selection"=w650:string)  [unwired: 17 in, 2 out]
        n353 = Bundle By Name(cluster=w653, "Field Selection"=w650) -> (w651:T8)
      }
      frame "Run Next Sequence" {
        n354 = Unbundle By Name(w655) -> ("Field Selection"=w660:string, "Auton Sequence"=w663:T3[], "Simulation Index"=w662:i32)
        n355 = Index Array(array=w663, index=w662) -> (element=w661:T3)
        n356 = Unbundle(w661) -> ("Sequence Array"=w659:T4[])
        n357 = for {
          tunnel: w659 -> [w669] mode=indexing
          tunnel: w660 -> [w673]
          tunnel: w658 -> [w670]
          tunnel: [w668] -> w656 if=w665
          tunnel: w655 -> [w667]
          tunnel: [w665] -> w657 if=w665
          n358 = Unbundle By Name(w669) -> ("Plate Arrangement"=w674:T2, "Command Name"=w672:string, "Data"=w671:variant)
          n359 = call "Plate Assignment Parse.vi"("Game String"=w673, "Plate Arrangement"=w674) -> ("Match?"=w666:bool)  [unwired: 9 in]
          n360 = case shown="True" w666 {
            tunnel: w672 -> [_ w682]
            tunnel: w671 -> [_ w681]
            tunnel: w670 -> [_ w680]
            tunnel: w669 -> [_ w679]
            tunnel: [w675 w678] -> w668
            tunnel: w667 -> [w675 w677]
            tunnel: [_ w676] -> w665
            frame False {
            }
            frame True {
              n361 = case shown="\"Drive Path\"" w682 {
                tunnel: w681 -> [_ _]
                tunnel: w680 -> [_ w691]
                tunnel: w679 -> [_ w689]
                tunnel: [w683 w688] -> w678
                tunnel: w677 -> [w683 w687]
                tunnel: [_ TRUE] -> w676
                frame Default {
                }
                frame "Drive Path" {
                  n362 = Bundle By Name(cluster=w687, "Current Command"=w689, "Sim Robot Index"=0) -> (w688:T8)
                  n363 = call "Enqueue Multiple.vi"("In Front? (F)"=TRUE, "Array"=string[] ["Sim Tick"], "Queue in"=w691) -> ()  [unwired: 7 in, 2 out]
                }
              }
            }
          }
        }
        n364 = Select(t=w656, s=w657, f=w655) -> (s? t:f=w654:T8)
      }
      frame "Sim Tick" {
        w705 = 5 ("Sim Speed")
        n365 = Unbundle By Name(w725) -> ("Sim Robot Index"=w714:i32, "Current Command"=w724:T4, "Field Half"=w717:cluster{dbl[], dbl[]}[], "Robot Index"=w718:i32)
        n366 = Unbundle By Name(w724) -> ("Data"=w723:variant)
        n367 = Index Array(array=w717, index=w718) -> (element=w719:cluster{dbl[], dbl[]})
        n368 = Get Variant Attribute(Variant=w723, name="_graphPlot", default value (empty Variant)=w719) -> (value=w721:cluster{dbl[], dbl[]})  [unwired: 1 in, 3 out]
        n369 = Unbundle(w721) -> (w701:dbl[], w715:dbl[])
        n370 = Array Size(array=w701) -> (size(s)=w700:i32)
        n371 = Array Subset(array=w701, index=w714, length=w705) -> (w710:dbl[])
        n372 = Array Subset(array=w715, index=w714, length=w705) -> (w709:dbl[])
        n373 = Decrement(x=w700) -> (x-1=w697:i32)
        n374 = call <vilib>:"Linear Fit.vi"("Y"=w709, "X"=w710) -> ("slope"=w708:dbl)  [unwired: 9 in, 4 out]
        n375 = Add(x=w714, y=w705) -> (x+y=w699:i32)
        n376 = Inverse Tangent(1:w708) -> (0:w694:dbl)
        n377 = In Range and Coerce(upper limit=w697, x=w699, lower limit=0) -> (coerced(x)=w696:i32, In Range?=w693:bool)
        n378 = case shown="True" w693 {
          tunnel: "Redraw Robot" -> [w728 w731]
          tunnel: "Sim Tick" -> [_ w730]
          tunnel: [w727 w729] -> w702
          frame False {
            n379 = Build Array(w728) -> (w727:string[])
          }
          frame True {
            n380 = Build Array(w731, w730) -> (w729:string[])
          }
        }
        n381 = Index Array(array=w701, index=w696) -> (element=w712:dbl)
        n382 = Index Array(array=w715, index=w696) -> (element=w713:dbl)
        n383 = Bundle("x"=w712, "y"=w713) -> (w711:cluster{"x":dbl, "y":dbl})  [unwired: 1 in]
        n384 = call "Enqueue Multiple.vi"("In Front? (F)"=TRUE, "Array"=w702, "Queue in"=w707) -> ()  [unwired: 7 in, 2 out]
        n385 = feedback-in #9(w694) -> ()
        n386 = feedback #9() -> (w695:dbl)  [unwired: 1 in]
        n387 = Select(t=w694, s=w693, f=w695) -> (s? t:f=w692:dbl)
        n388 = Bundle By Name(cluster=w725, "Sim Robot Index"=w696, "Robot Position"=w711, "Theta"=w692) -> (w720:T8)
        n389 = Wait (ms)(milliseconds to wait=u32 100) -> ()  [unwired: 1 out]
      }
      frame "Sequence Next" {
        n390 = Unbundle By Name(w739) -> ("Auton Sequence"=w738:T3[], "Simulation Index"=w737:i32)
        n391 = Array Size(array=w738) -> (size(s)=w735:i32)
        n392 = Increment(x=w737) -> (x+1=w733:i32)
        n393 = Greater?(x=w735, y=w733) -> (0:w734:bool)
        n394 = case shown="True" w734 {
          tunnel: w732 -> [w741 w742]
          frame False {
            n395 = Flush Queue(queue=w741) -> ()  [unwired: 1 in, 3 out]
          }
          frame True {
            n396 = call "Enqueue Multiple.vi"("Array"=string[] ["Run Next Sequence", "Sequence Next"], "Queue in"=w742) -> ()  [unwired: 8 in, 2 out]
            n397 = Wait (ms)(milliseconds to wait=u32 500) -> ()  [unwired: 1 out]
          }
        }
        n398 = Bundle By Name(cluster=w739, "Simulation Index"=w733) -> (w736:T8)
      }
      frame "/**** File Operations ****/" {
      }
      frame "Save File" {
        n399 = Unbundle By Name(w758) -> ("Active Path"=w753:path, "Auton Sequence"=w752:T3[], "y position"=w749:dbl)
        n400 = To Variant(anything=w752) -> (Variant=w750:variant)
        n401 = Set Variant Attribute(Variant=w750, name="y position", value=w749, error in=w756) -> (Variant out=w747:variant, error out=w751:errorcluster)  [unwired: 1 out]
        n402 = Write to Binary File(file (use dialog)=w753, data=w747, error in=w751) -> (refnum out=w754:refnum<file>, error out=w755:errorcluster)  [unwired: 3 in, 1 out]
        n403 = Close File(refnum=w754, error in=w755) -> (error out=w757:errorcluster)  [unwired: 1 out]
      }
      frame "Open File" {
        n404 = Unbundle By Name(w777) -> ("Auton Sequence"=w769:T3[], "Active Path"=w771:path)
        n405 = Read from Binary File(5:variant, 8:w772, 10:-1 ("count (1)"), 11:w771) -> (0:w775:errorcluster, 2:w765:variant[], 3:w774:refnum<file>)  [unwired: 2 in, 1 out]
        n406 = Close File(refnum=w774, error in=w775) -> (error out=w768:errorcluster)  [unwired: 1 out]
        n407 = Index Array(array=w765) -> (element=w764:variant)  [unwired: 1 in]
        n408 = Variant To Data(error in=w768, type=w769, Variant=w764) -> (data=w767:T3[], error out=w766:errorcluster)
        n409 = Get Variant Attribute(Variant=w764, name="y position", default value (empty Variant)=0.0, error in=w766) -> (value=w761:dbl, error out=w760:errorcluster)  [unwired: 2 out]
        n410 = case shown="No Error" w760 {
          tunnel: w777 -> [w784 w785]
          tunnel: [w783 w785] -> w773
          tunnel: w767 -> [w782 _]
          tunnel: w761 -> [w781 _]
          tunnel: w759 -> [w778 _]
          frame No Error {
            n411 = Bundle By Name(cluster=w784, "Auton Sequence"=w782, "y position"=w781, "Load Index"=0) -> (w783:T8)
            n412 = call "Enqueue Multiple.vi"("Array"=string[] ["Adjust Field", "Build Field", "Add Robot", "Reload Listbox", "Reload Graphs", "Check Auton Sequence"], "Queue in"=w778) -> ()  [unwired: 8 in, 2 out]
          }
          frame Error {
          }
        }
      }
      frame "Reload Graphs" {
        n413 = Unbundle By Name(w791) -> ("Field Half"=w789:cluster{dbl[], dbl[]}[], "Auton Sequence"=w790:T3[])
        n414 = for {
          tunnel: w790 -> [w798] mode=indexing
          shift-right: [w795] -> w787
          shift-left: w789 -> [w796]
          tunnel: [w793] -> w786 mode=indexing
          n415 = Unbundle(w798) -> ("Sequence Array"=w797:T4[])
          n416 = for {
            tunnel: w797 -> [w803] mode=indexing
            shift-right: [w806] -> w795
            shift-left: w796 -> [w800]
            tunnel: [w801] -> w794 mode=indexing
            n417 = Unbundle By Name(w803) -> ("Data"=w811:variant)
            n418 = Array Size(array=w800) -> (size(s)=w799:i32)
            n419 = Get Variant Attribute(Variant=w811, name="_graphPlot", default value (empty Variant)=cluster{dbl[], dbl[]} {[], []} ("element")) -> (duplicate Variant=w805:variant, found=w808:bool, value=w807:cluster{dbl[], dbl[]})  [unwired: 1 in, 1 out]
            n420 = case shown="True" w808 {
              tunnel: w800 -> [w813 w820]
              tunnel: w807 -> [_ w818]
              tunnel: [w813 w819] -> w806
              tunnel: w805 -> [w812 w817]
              tunnel: "_graphIndex" ("name") -> [_ w816]
              tunnel: [w812 w815] -> w802
              tunnel: w799 -> [_ w814]
              frame False {
              }
              frame True {
                n421 = Set Variant Attribute(Variant=w817, name=w816, value=w814) -> (Variant out=w815:variant)  [unwired: 1 in, 2 out]
                n422 = Build Array (concatenate)(w820, w818) -> (w819:cluster{dbl[], dbl[]}[])
              }
            }
            n423 = Bundle By Name(cluster=w803, "Data"=w802) -> (w801:T4)
          }
          n424 = Bundle(w794) -> (w793:cluster{T4[]})  [unwired: 1 in]
        }
        n425 = Bundle By Name(cluster=w791, "Field Half"=w787, "Auton Sequence"=w786) -> (w788:T8)
      }
      frame "Reload Listbox" {
        n426 = Unbundle By Name(w822) -> ("Auton Sequence"=w821:T3[])
        n427 = control-ref of="Sequence"() -> (w823:refnum<vi>)
        n428 = call "Update Table Display.vi"("Auton Sequence"=w821, "MulticolumnListbox in"=w823) -> ()  [unwired: 10 in]
      }
    }
    n429 = Unbundle By Name(w26) -> ("Field Half"=→"Field Half":cluster{dbl[], dbl[]}[], "Current Command.Command Name"=→"Current Command":string, "Auton Sequence"=w22:T3[])
    n430 = local write "Auton Sequence"(w22) -> ()
  }
  n431 = disable-structure shown="Enabled" {
    disable-tunnel: _ -> [w825 _]
    frame Disabled {
      n432 = for {
        tunnel: w825 -> [w828] mode=indexing
        n433 = Unbundle(w828) -> ("Sequence Array"=w826)
        n434 = Array Size(array=w826) -> (size(s)=w827:i32)
        n435 = for {
          tunnel: w826 -> [w837]
          workers-P: w827 -> [_]
          n436 = Unbundle By Name(w837) -> ("Command Name"=w833, "Data"=w835)  [unwired: 1 out]
          n437 = Open VI Reference(vi path=w833) -> (vi reference=w836:refnum<vi>)  [unwired: 5 in, 1 out]
          n438 = invoke class="VI" method="Ctrl Val.Set"(reference=w836, "Control Name"="Data", "Value"=w835) -> (reference out=w832:refnum<vi>)  [unwired: 2 in, 4 out]
          n439 = invoke class="VI" method="Run VI"(reference=w832, "Wait until done"=TRUE ("Wait Until Done"), "Auto Dispose Ref"=FALSE ("Auto Dispose Reference")) -> (reference out=w831:refnum<vi>)  [unwired: 2 in, 4 out]
          n440 = Close Reference(reference=w831) -> ()  [unwired: 1 in, 1 out]
        }
      }
    }
    frame Enabled {
    }
  }
